vi "ML SAM3 test.vi"() -> ()   [LabVIEW 2022 SP3]
uses:
  <vilib>/httpClient/POSTBuffer.vi
  <vilib>/httpClient/LabVIEWHTTPClient.lvlib
  <vilib>/vision/Image Controls.llb/IMAQ Image.ctl
panel:
  in  "Image":T1
  out "error out":errorcluster
  out "headers":string
  out "body":string
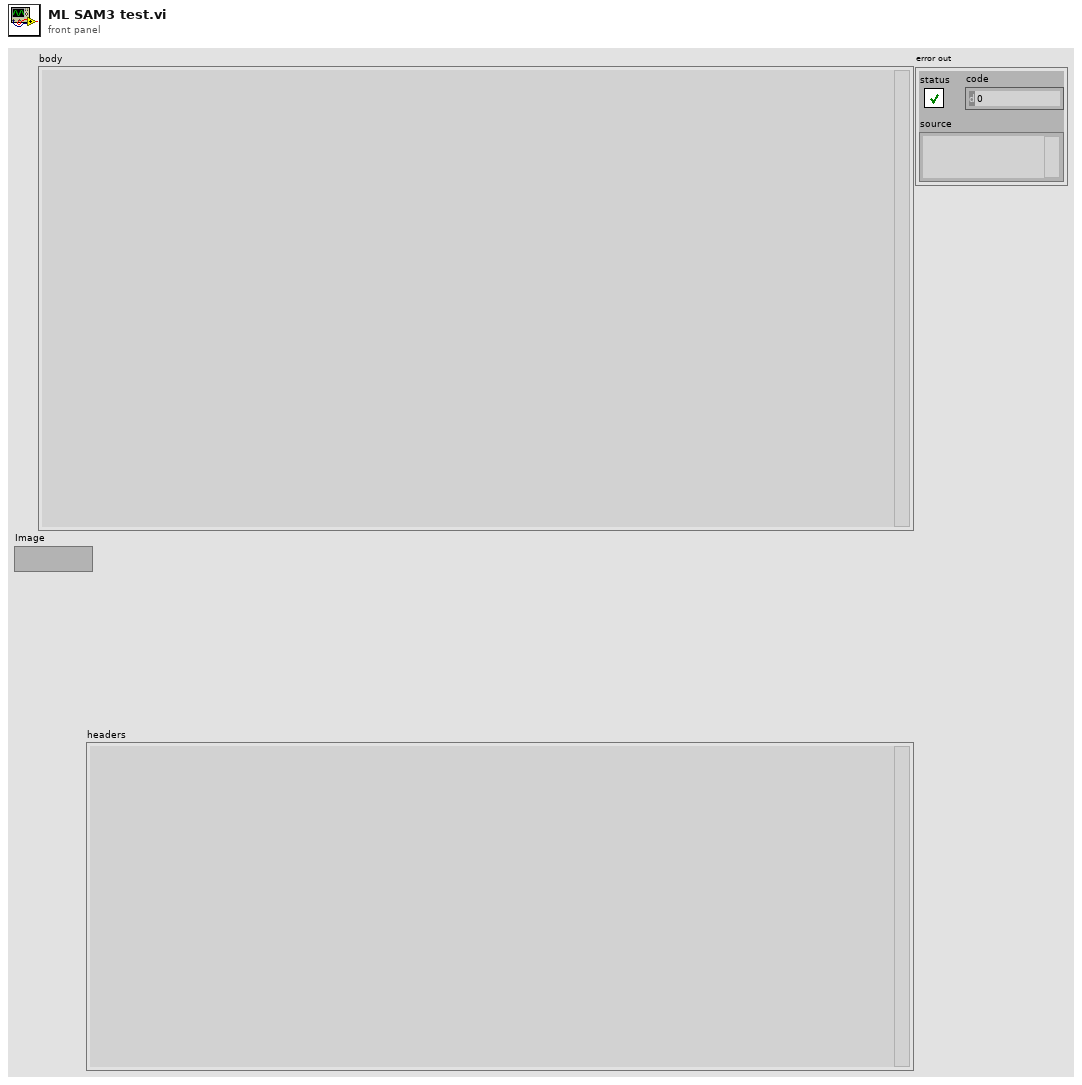
[diagram p1: front panel]
types:
  T1 = typedef "IMAQ Image.ctl" = refnum<image>
  T2 = typedef "LabVIEWHTTPClient.lvlib/ClientHandle.ctl" = refnum<k1>
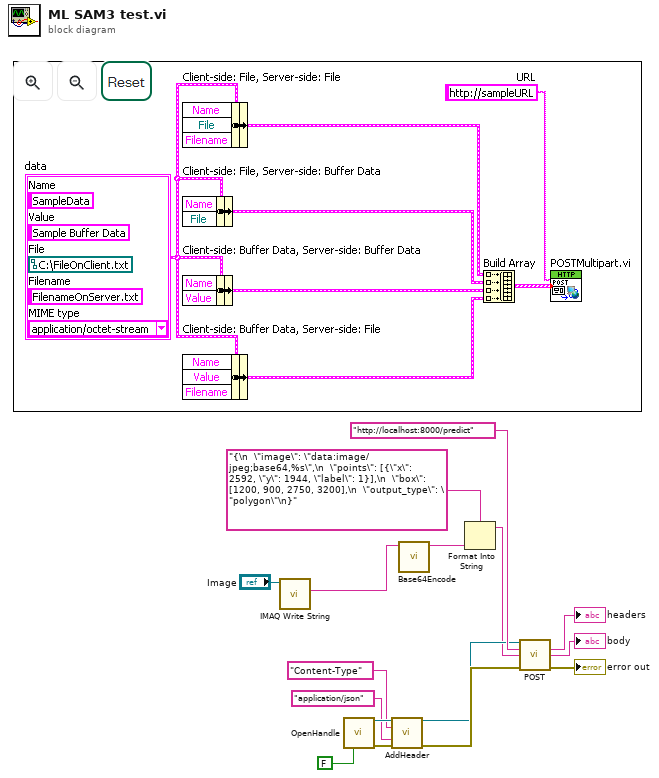
[diagram p0: block diagram]
diagram:
  n1 = call-poly "IMAQ Write String"("Image"="Image") -> ("FileString"=w2:string)  [unwired: 8 in, 2 out]
  n2 = call <vilib>:"OpenHandle.vi"("verify server(true)"=FALSE) -> ("client handle out"=w9:T2, "error out"=w16:errorcluster)  [unwired: 13 in]
  n3 = call <vilib>:"AddHeader.vi"("client handle"=w9, "header"="Content-Type", "value"="application/json", "error in (no error)"=w16) -> ("client handle out"=w8:T2, "error out"=w10:errorcluster)  [unwired: 10 in]
  n4 = call <vilib>:"Base64Encode.vi"("buffer in"=w2) -> ("encoded string"=w4:string)  [unwired: 9 in, 1 out]
  n5 = Format Into String(format string="{\n  \"image\": \"data:image/jpeg;base64,%s\",\n  \"points\": [{\"x\": 2592, \"y\": 1944, \"label\": 1}],\n  \"box\": [1200, 900, 2750, 3200],\n  \"output_type\": \"polygon\"\n}", w4) -> (resulting string=w3:string)  [unwired: 2 in, 1 out]
  n6 = call-poly <vilib>:"POST.vi"("client handle"=w8, "url"="http://localhost:8000/predict", "buffer"=w3, "error in (no error)"=w10) -> ("headers"=→"headers":string, "body"=→"body":string, "error out"=→"error out":errorcluster)  [unwired: 8 in, 1 out]
